vi "Simulation Initialize.vi"(0 "simulation configuration":T1={"maxTime"=5.0, "enableVisualization"=TRUE, "statechart"=path "iRobot Navigation State Machine.vi", "environment"=path "iRobot Navigation State Machine.vi", "record"=path "Simulation Record.xml", "autograde?"=TRUE, "interactive?"=FALSE, "feedback mode"=enum."debug navigation"}, 2 "Statechart display":refnum<vi>, 3 "Simulator display":refnum<vi>, 11 "Error In":errorcluster) -> (4 "simulator":T3={"configuration"={"maxTime"=5.0, "enableVisualization"=TRUE, "statechart"=path "iRobot Navigation State Machine.vi", "environment"=path "iRobot Navigation State Machine.vi", "record"=path "Simulation Record.xml", "autograde?"=TRUE, "interactive?"=FALSE, "feedback mode"=enum."debug navigation"}, "Bump Sensors"=[], "Distance Sensors"=[], "Accelerometer"=refnum, "Wall Sensor"=refnum, "Statechart\ndisplay"=refnum, "Body"=refnum, "Left Motor"=refnum, "Right Motor"=refnum, "first step?"=FALSE}, 15 "Error Out":errorcluster)   [LabVIEW 2014]
uses:
  Simulator.ctl
  <instrlib>/DC Motor Controller/HAIOL/DC Motor Controller.lvclass
  CyberSim interface/Simulation Configuration.ctl
  autograder/feedbackMode.ctl
  <vilib>/Robotics/Simulator/Engine/ctl/Simulation Mode.ctl
  <vilib>/Robotics/Simulator/Engine/ctl/Step Mode.ctl
  Simulation Trace Operation.ctl
  Simulation Call Statechart Operation.ctl
  <vilib>/robotics/Simulator/NI_Robotics_Simulator.lvlib
panel:
  out "error out":errorcluster
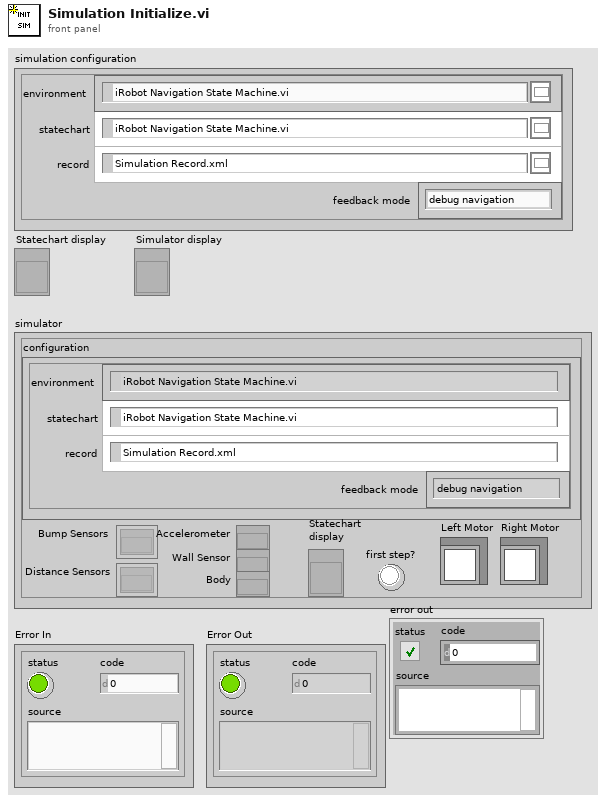
[diagram p1: front panel]
types:
  T1 = typedef "Simulation Configuration.ctl" = cluster{"maxTime":sgl, "enableVisualization":bool, "statechart":path, "environment":path, "record":path, "autograde?":bool, "interactive?":bool, "feedback mode":T2}
  T2 = typedef "feedbackMode.ctl" = enum32{"debug navigation", "debug hill climb", "autograde navigation", "autograde hill climb"}
  T3 = typedef "Simulator.ctl" = cluster{"configuration":T1, "Bump Sensors":refnum<k20>[], "Distance Sensors":refnum<k20>[], "Accelerometer":refnum<k20>, "Wall Sensor":refnum<k20>, "Statechart\ndisplay":refnum<vi>, "Body":refnum<k20>, "Left Motor":refnum<class "DC Motor Controller.lvclass">, "Right Motor":refnum<class "DC Motor Controller.lvclass">, "first step?":bool}
  T4 = typedef "Simulation Call Statechart Operation.ctl" = enum16{"Initialize", "Call Statechart", "Finalize"}
  T5 = typedef "Simulation Trace Operation.ctl" = enum16{"Initialize", "Record Trace Element", "Get Trace"}
  T6 = typedef "NI_Robotics_Simulator.lvlib/Step Mode.ctl" = u16
  T7 = typedef "NI_Robotics_Simulator.lvlib/Simulation Mode.ctl" = u16
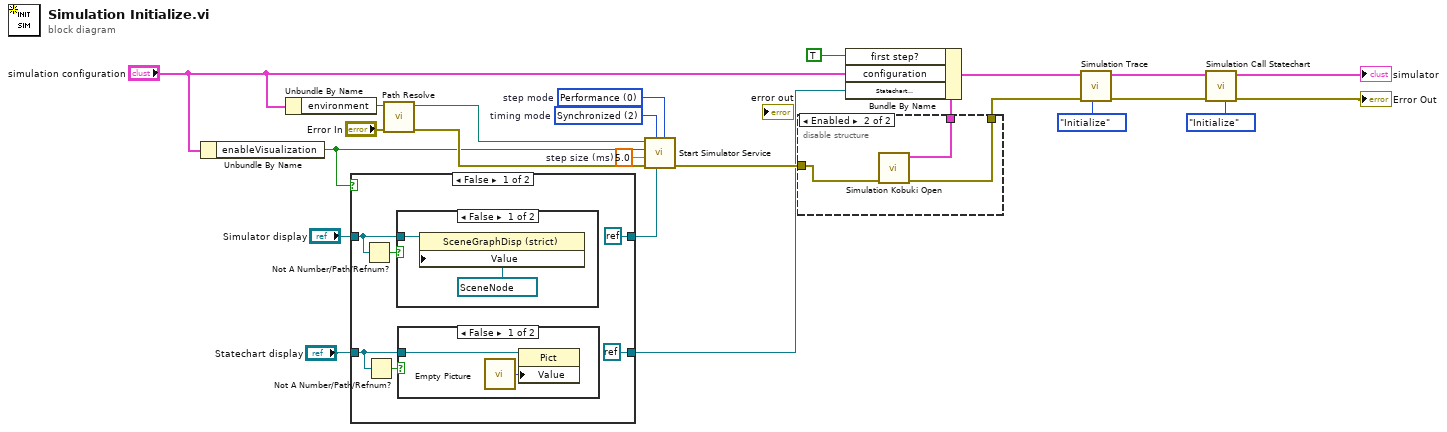
[diagram p0: block diagram]
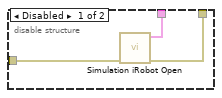
[diagram p2: hidden frame]
diagram:
  w14 = 5.0  # step size (ms)
  w23 = T6 0 items=["Performance", "Accuracy"]  # step mode
  w24 = T7 2 items=["Software Real-Time", "Free Running", "Synchronized"]  # timing mode
  n1 = Unbundle By Name("simulation configuration") -> ("enableVisualization"=w10:bool)
  n2 = Unbundle By Name("simulation configuration") -> ("environment"=w18:path)
  n3 = case shown="False" w10 {
    tunnel: "Simulator display" -> [w28 w36]
    tunnel: [refnum<k0> refnum w36] -> w8
    tunnel: "Statechart display" -> [w26 w35]
    tunnel: [refnum<k0> refnum w35] -> w6
    frame False {
      n4 = Not A Number/Path/Refnum?(number/path/refnum=w28) -> (NaN/Path/Refnum?=w29:bool)
      n5 = Not A Number/Path/Refnum?(number/path/refnum=w26) -> (NaN/Path/Refnum?=w27:bool)
      n6 = case shown="False" w29 {
        tunnel: w28 -> [w34 _]
        frame False {
          n7 = property class="SceneGraphDisp (strict)"(reference=w34, "Value"=refnum<vi> refnum ("3D Picture")) -> ()  [unwired: 1 in, 2 out]
        }
        frame True {
        }
      }
      n8 = case shown="False" w27 {
        tunnel: w26 -> [w32 _]
        frame False {
          n9 = call "Empty Picture"() -> ("empty picture"=w31:picture)
          n10 = property class="Pict"(reference=w32, "Value"=w31) -> ()  [unwired: 1 in, 2 out]
        }
        frame True {
        }
      }
    }
    frame True {
    }
  }
  n11 = call "Path Resolve.vi"("Error In"="Error In", "absolute or relative path"=w18) -> ("Error Out"=w17:errorcluster, "resolved path"=w1:path)  [unwired: 8 in]
  n12 = call <vilib>:"Start Simulator Service.vi"("step mode"=w23, "3D picture refnum"=w8, "timing mode"=w24, "error in (no error)"=w17, "step size (ms)"=w14, "enable 3D visualization (T)"=w10, "manifest file"=w1) -> ("error out"=w21:errorcluster)  [unwired: 4 in]
  n13 = disable-structure shown="Enabled" {
    disable-tunnel: [w39 w41] -> w22
    disable-tunnel: w21 -> [w38 w42]
    disable-tunnel: [w37 w40] -> w15
    frame Disabled {
      n14 = call "Simulation iRobot Open.vi"("error in (no error)"=w38) -> ("error out"=w37:errorcluster, "simulator"=w39:T3)  [unwired: 8 in, 1 out]
    }
    frame Enabled {
      n15 = call "Simulation Kobuki Open.vi"("error in (no error)"=w42) -> ("error out"=w40:errorcluster, "simulator"=w41:T3)  [unwired: 8 in, 1 out]
    }
  }
  n16 = Bundle By Name(cluster=w22, "first step?"=TRUE, "configuration"="simulation configuration", "Statechart\ndisplay"=w6) -> (w16:T3)
  n17 = call "Simulation Trace.vi"("operation"=Simulation_Trace_Operation."Initialize", "error in"=w15, "simulator"=w16) -> ("error out"=w12:errorcluster, "simulator"=w13:T3)  [unwired: 5 in, 2 out]
  n18 = call "Simulation Call Statechart.vi"("operation"=Simulation_Call_Statechart_Operation."Initialize", "error in"=w12, "simulator"=w13) -> ("error out"=→"Error Out":errorcluster, "simulator"=→"simulator":T3)  [unwired: 6 in, 1 out]
